vi "ZK仪器状态.vi"(7 "运行模式":string, 8 "error in (no error)":errorcluster, 11 "Slave ID":T3) -> (0 "error out":errorcluster, 2 "质控仪器状态显示":T1, 3 "质控仪器状态":T2 {"当前步骤数" format="0x%04xH"})   [LabVIEW 2016, in "质控单元V4.lvlib"]
uses:
  <vilib>/Plasmionique/MB Master/MB_Master/MB_Master.lvclass
  <vilib>/Plasmionique/MB Master/MB Master.lvlib
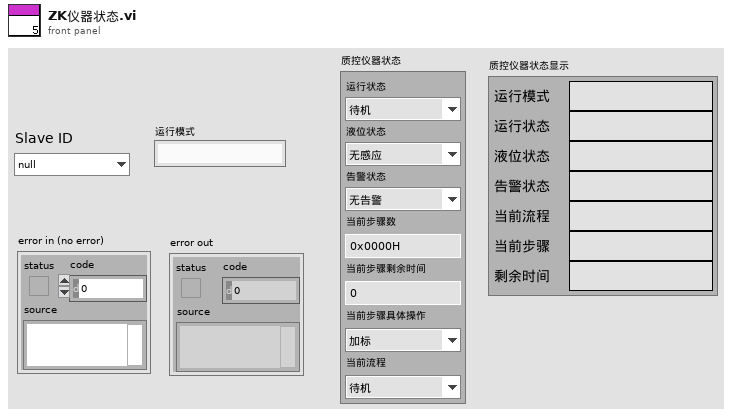
[diagram p1: front panel]
types:
  T1 = typedef "质控单元V4.lvlib/质控仪器状态显示.ctl" = cluster{"运行模式":string, "运行状态":string, "液位状态":string, "告警状态":string, "当前流程":string, "当前步骤":string, "剩余时间":string}
  T2 = typedef "质控单元V4.lvlib/质控仪器状态.ctl" = cluster{"运行状态":enum16{"待机", "润洗", "进样", "定量", "加标", "等待取样", "排液", "异常停机"}, "液位状态":enum16{"无感应", "有感应"}, "告警状态":enum16{"无告警", "液位故障告警", "注射泵异常"}, "当前步骤数":u16, "当前步骤剩余时间":u16, "当前步骤具体操作":enum16{"加标", "进样", "排液", "搅拌", "定量"}, "当前流程":enum16{"待机", "进样流程", "加标流程", "排液流程", "水样润洗流程", "加标润洗流程"}}
  T3 = typedef "质控单元V4.lvlib/质控slave id.ctl" = enum16{"null", "氨氮", "总磷", "总氮", "CODMn", "CODCr", "氟化物", "挥发酚"}
  T4 = cluster{"Registers[0]":u16, "Registers[1]":u16, "Registers[2]":u16, "Registers[3]":u16, "Registers[4]":u16, "Registers[5]":u16, "Registers[6]":u16}
  T5 = enum16{"待机", "润洗", "进样", "定量", "加标", "等待取样", "排液", "异常停机"}
  T6 = cluster{"运行模式":string, "RingText.Text":string, "RingText.Text":string, "RingText.Text":string, string, "RingText.Text":string, string}
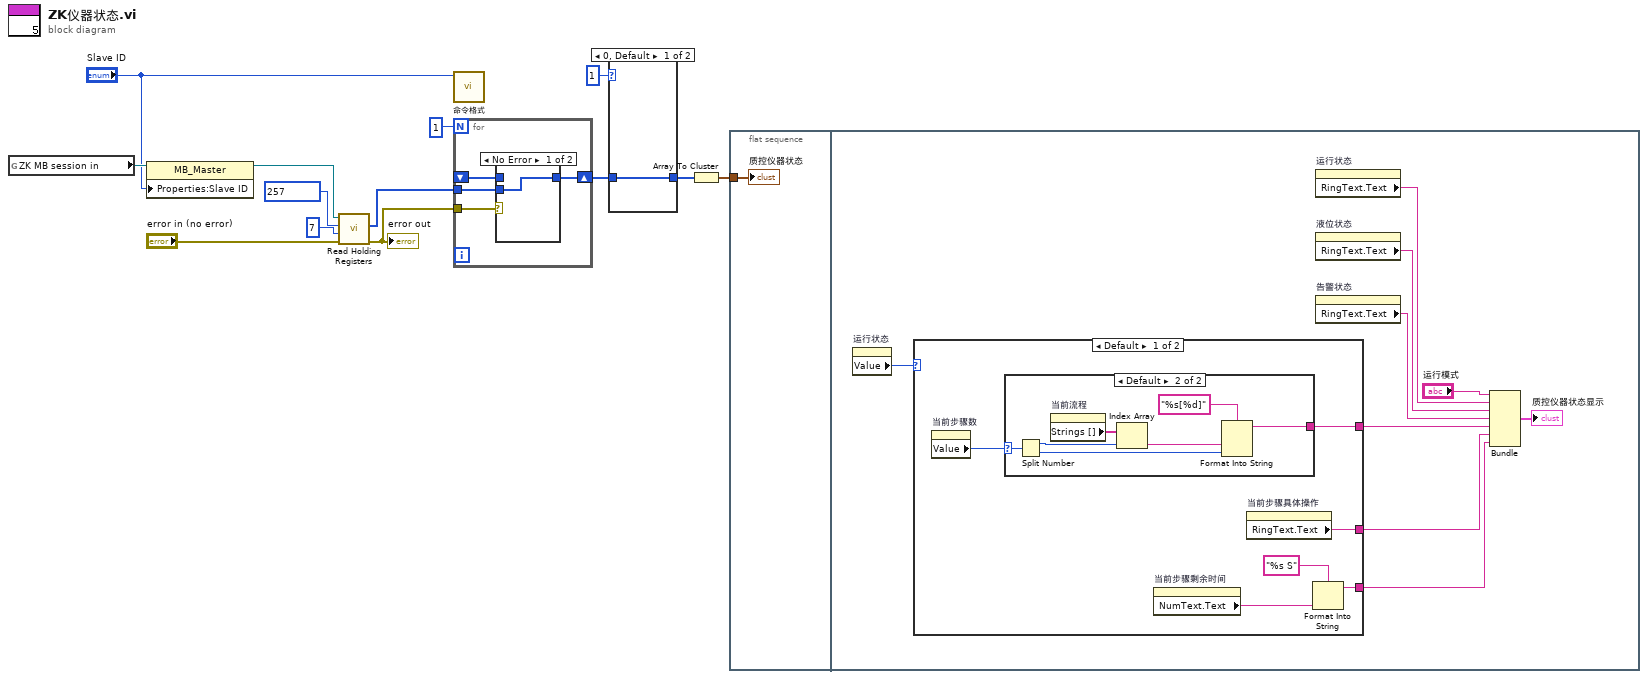
[diagram p0: block diagram]
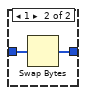
[diagram p2: hidden frame]
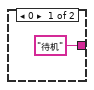
[diagram p3: hidden frame]
diagram:
  n1 = global read "ZK非断电保存全局变量.vi" "ZK MB session in"() -> (w12:refnum<class "MB_Master.lvclass">)
  n2 = property class="MB_Master"(reference=w12, "Properties:Slave ID"="Slave ID") -> (reference out=w10:refnum<class "MB_Master.lvclass">)  [unwired: 1 in, 1 out]
  n3 = call <vilib>:"Read Holding Registers.vi"("error in (no error)"="error in (no error)", "quantity"=u16 7, "starting address"=u16 257, "MB session in"=w10) -> ("error out"=w7:errorcluster, "Registers"=w6:u16[])  [unwired: 5 in, 1 out]
  "error out" <- w7
  n4 = call "命令格式.vi"("站号"="Slave ID") -> ()  [unwired: 10 in, 1 out]
  n5 = for {
    N: 1 -> [_]
    tunnel: w7 -> [w17]
    tunnel: w6 -> [w16]
    shift-right: [w15] -> w5
    shift-left: _ -> [w14]
    n6 = case shown="No Error" w17 {
      tunnel: w16 -> [w18 _]
      tunnel: [w18 w19] -> w15
      tunnel: w14 -> [_ w19]
      frame No Error {
      }
      frame Error {
      }
    }
  }
  n7 = case shown="0, Default" u16 1 ("命令格式") {
    tunnel: w5 -> [w20 w22]
    tunnel: [w20 w21] -> w4
    frame 0, Default {
    }
    frame 1 {
      n8 = Swap Bytes(anything=w22) -> (byte swapped=w21:u16[])
    }
  }
  n9 = Array To Cluster(array=w4) -> (cluster=w3:T4)
  n10 = flat-sequence {
    tunnel: w3 -> [w23]
    frame #0 {
      "质控仪器状态" <- w23
    }
    frame #1 {
      n11 = property on="运行状态" class="Enum (strict)"() -> ("Value"=w25:T5)  [unwired: 2 in, 2 out]
      n12 = case shown="Default" w25 {
        tunnel: [w38 _] -> w29
        tunnel: [w37 _] -> w28
        tunnel: [w34 _] -> w27
        frame Default {
          n13 = property on="当前步骤数" class="DigNum (strict)"() -> ("Value"=w33:u16)  [unwired: 2 in, 2 out]
          n14 = case shown="Default" w33 {
            selector: w33 -> [_ w40]
            tunnel: ["待机" w41] -> w38
            frame 0 {
            }
            frame Default {
              n15 = Split Number(x=w40) -> (hi(x)=w45:u8, lo(x)=w43:u8)
              n16 = property on="当前流程" class="Enum (strict)"() -> ("Strings []"=w44:string[])  [unwired: 2 in, 2 out]
              n17 = Index Array(array=w44, index=w45) -> (element=w46:string)
              n18 = Format Into String(format string="%s[%d]" ("格式字符串"), w46, w43) -> (resulting string=w41:string)  [unwired: 2 in, 1 out]
            }
          }
          n19 = property on="当前步骤剩余时间" class="DigNum (strict)"() -> ("NumText.Text"=w35:string)  [unwired: 2 in, 2 out]
          n20 = property on="当前步骤具体操作" class="Enum (strict)"() -> ("RingText.Text"=w37:string)  [unwired: 2 in, 2 out]
          n21 = Format Into String(format string="%s S" ("格式字符串"), w35) -> (resulting string=w34:string)  [unwired: 2 in, 1 out]
        }
        frame "待机", "等待取样" {
        }
      }
      n22 = property on="运行状态" class="Enum (strict)"() -> ("RingText.Text"=w32:string)  [unwired: 2 in, 2 out]
      n23 = property on="液位状态" class="Enum (strict)"() -> ("RingText.Text"=w31:string)  [unwired: 2 in, 2 out]
      n24 = property on="告警状态" class="Enum (strict)"() -> ("RingText.Text"=w30:string)  [unwired: 2 in, 2 out]
      n25 = Bundle("运行模式"="运行模式", "RingText.Text"=w32, "RingText.Text"=w31, "RingText.Text"=w30, w29, "RingText.Text"=w28, w27) -> (→"质控仪器状态显示":T6)  [unwired: 1 in]
    }
  }
